vi "get Session Prefix.vi"(7 "Session - Root":refnum<class "Sequence Automation Session.lvclass">) -> (8 "Session Prefix":string)   [LabVIEW 2018, in "Sequence Automation Session.lvlib" / "Sequence Automation Session.lvclass"]
uses:
  Sequence Automation Session.lvclass
  Sequence Automation Session.lvclass/Sequence Automation Session.ctl
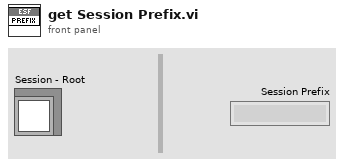
[diagram p1: front panel]
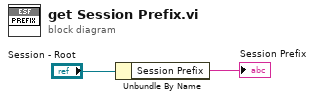
[diagram p0: block diagram]
diagram:
  n1 = Unbundle By Name("Session - Root") -> ("Session Prefix"=→"Session Prefix":string)
